vi "SwerveKinematics_NormalizeChassisSpeeds.vi"(7 "in SWERVE_DRIVE_KINEMATICS":T1 {"SavedModuleStates"."Angle"."SIN" format="%13.4f"; "SavedModuleStates"."Angle"."COS" format="%13.4f"; "SavedModuleStates"."Angle"."VALUE" format="%13.4f"; "PrevCoR"."Y" format="%14.3f"; "PrevCoR"."X" format="%14.3f"; "Modules"."Y" format="%14.3f"; "Modules"."X" format="%14.3f"}, 9 "AttainableMaxSpeed":dbl, 11 "in Chassis Speed":T6 {"vOmega" format="%10.3f"; "vY" format="%10.3f"; "vX" format="%10.3f"}) -> (3 "out Chassis Speed":T6 {"vOmega" format="%10.3f"; "vY" format="%10.3f"; "vX" format="%10.3f"}, 5 "out SWERVE_DRIVE_KINEMATICS":T1 {"SavedModuleStates"."Angle"."SIN" format="%13.4f"; "SavedModuleStates"."Angle"."COS" format="%13.4f"; "SavedModuleStates"."Angle"."VALUE" format="%13.4f"; "PrevCoR"."Y" format="%14.3f"; "PrevCoR"."X" format="%14.3f"; "Modules"."Y" format="%14.3f"; "Modules"."X" format="%14.3f"})   [LabVIEW 2019, in "Trajectory_Library.lvlib"]
doc: "Normalizes the wheel speeds using some max attainable speed. Sometimes, after inverse kinematics, the requested speed from a/several modules may be above the max attainable speed for the driving motor on that module. To fix this issue, one can \"normalize\" all the wheel speeds to make sure that all requested module speeds are below the absolute threshold, while maintaining the ratio of speeds between modules.\n \nParameters:\n - moduleStates - Array of module states. \n - attainableMaxSpeed - The absolute max speed that a module can reach. (Meters/Sec)\n \n\nReturns:\n - out Wheel States -- Array of normalzied Wheel States"
uses:
  Trajectory_Library.lvlib
  TypeDef/CHASSIS_SPEEDS.ctl
  <vilib>/Analysis/Matrix/Datatypes/RealMatrix.ctl
  <vilib>/Analysis/Matrix/NI_Matrix.lvlib
  TypeDef/TRANSLATION2D.ctl
  TypeDef/ROTATION2D.ctl
  TypeDef/SWERVE_DRIVE_MODULE_STATE.ctl
  TypeDef/SWERVE_DRIVE_KINEMATICS.ctl
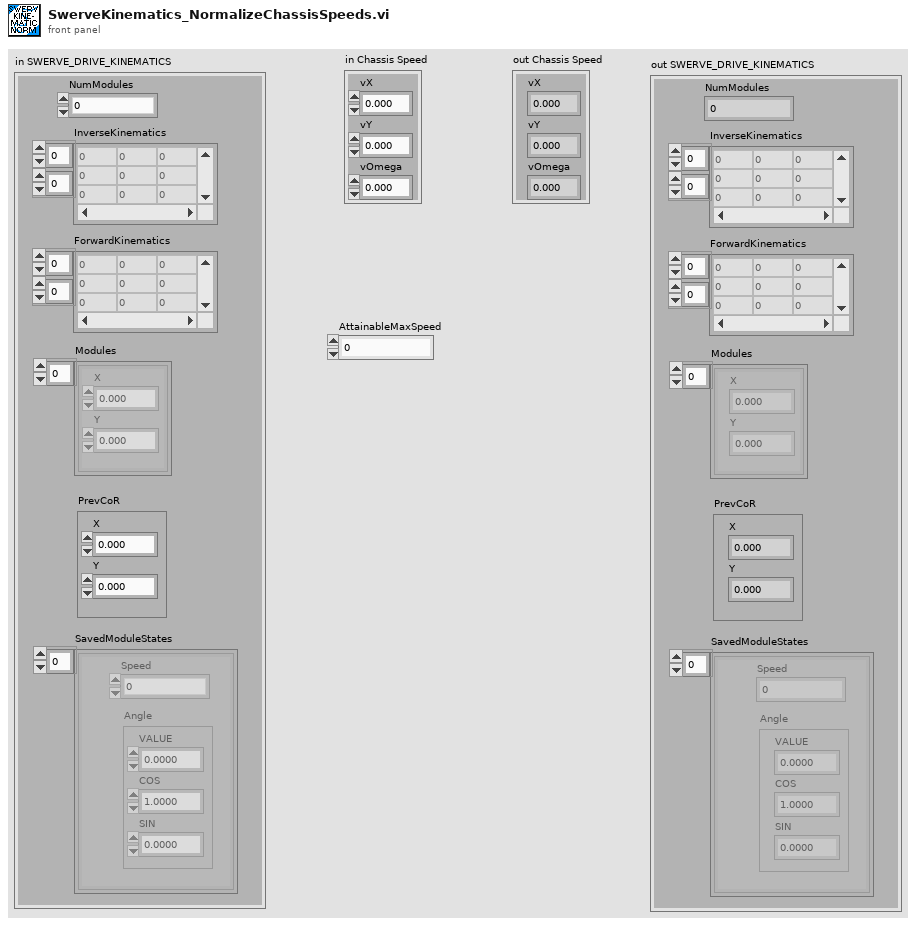
[diagram p1: front panel]
types:
  T1 = typedef "Trajectory_Library.lvlib/SWERVE_DRIVE_KINEMATICS.ctl" = cluster{"NumModules":i32, "InverseKinematics":T2, "ForwardKinematics":T2, "Modules":T3[], "PrevCoR":T3, "SavedModuleStates":T4[]}
  T2 = typedef "NI_Matrix.lvlib/RealMatrix.ctl" = dbl[][]
  T3 = typedef "Trajectory_Library.lvlib/TRANSLATION2D.ctl" = cluster{"X":dbl, "Y":dbl}
  T4 = typedef "Trajectory_Library.lvlib/SWERVE_DRIVE_MODULE_STATE.ctl" = cluster{"Speed":dbl, "Angle":T5}
  T5 = typedef "Trajectory_Library.lvlib/ROTATION2D.ctl" = cluster{"VALUE":dbl, "COS":dbl, "SIN":dbl}
  T6 = typedef "Trajectory_Library.lvlib/CHASSIS_SPEEDS.ctl" = cluster{"vX":dbl, "vY":dbl, "vOmega":dbl}
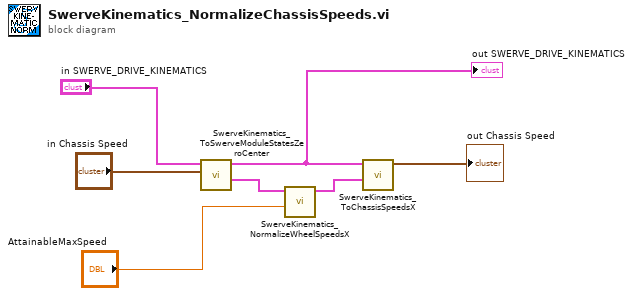
[diagram p0: block diagram]
diagram:
  n1 = call "SwerveKinematics_ToSwerveModuleStatesZeroCenter.vi"("ChassisSpeeds"="in Chassis Speed", "in SWERVE_DRIVE_KINEMATICS"="in SWERVE_DRIVE_KINEMATICS") -> ("ModuleStates"=w7:T4[], "out SWERVE_DRIVE_KINEMATICS"=w4:T1)  [unwired: 8 in]
  "out SWERVE_DRIVE_KINEMATICS" <- w4
  n2 = call "SwerveKinematics_NormalizeWheelSpeedsX.vi"("AttainableMaxSpeed"="AttainableMaxSpeed", "in WheelStates"=w7) -> ("out WheelStates"=w6:T4[])  [unwired: 9 in]
  n3 = call "SwerveKinematics_ToChassisSpeedsX.vi"("WheelStates"=w6, "in SWERVE_DRIVE_KINEMATICS"=w4) -> ("Chassis Speed"=→"out Chassis Speed":T6)  [unwired: 9 in]
